vi "Transform.vi"(8 "error in (no error)":errorcluster, 9 "Offset":u64, 10 "Transformation Map":refnum<class "Range.lvclass">, 11 "Range in":refnum<class "Range.lvclass">) -> (0 "error out":errorcluster, 2 "Remainder":refnum<class "Range.lvclass">, 3 "Range out":refnum<class "Range.lvclass">)   [LabVIEW 2020, in "Range.lvclass"]
uses:
  Range.lvclass
  Range.lvclass/Range.ctl
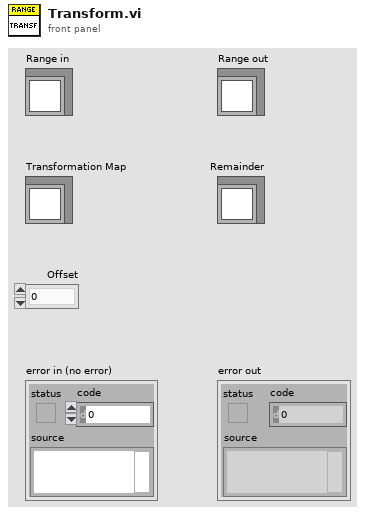
[diagram p1: front panel]
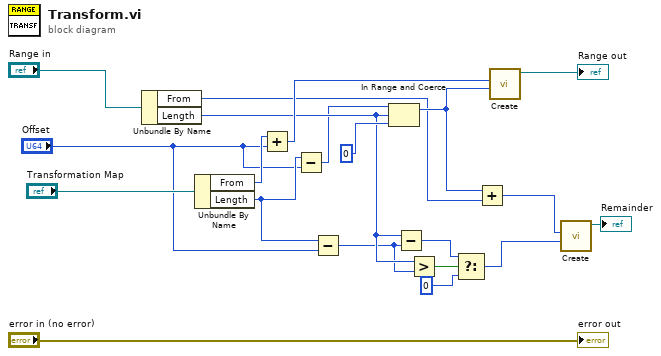
[diagram p0: block diagram]
diagram:
  n1 = Unbundle By Name("Range in") -> ("From"=w11:u64, "Length"=w8:u64)
  n2 = Unbundle By Name("Transformation Map") -> ("From"=w16:u64, "Length"=w13:u64)
  n3 = Add(x=w16, y="Offset") -> (x+y=w14:u64)
  n4 = Subtract(x=w13, y="Offset") -> (x-y=w2:u64)
  n5 = Subtract(x=w13, y="Offset") -> (x-y=w7:u64)
  n6 = In Range and Coerce(upper limit=w2, x=w8, lower limit=u64 0) -> (coerced(x)=w12:u64)  [unwired: 1 out]
  n7 = Subtract(x=w8, y=w7) -> (x-y=w5:u64)
  n8 = Greater?(x=w8, y=w7) -> (0:w6:bool)
  n9 = Select(t=w5, s=w6, f=u64 0) -> (s? t:f=w4:u64)
  n10 = Add(x=w12, y=w11) -> (x+y=w10:u64)
  n11 = call "Create.vi"("Length"=w12, "From"=w14) -> ("Range"=→"Range out":refnum<class "Range.lvclass">)  [unwired: 8 in, 1 out]
  n12 = call "Create.vi"("Length"=w4, "From"=w10) -> ("Range"=→"Remainder":refnum<class "Range.lvclass">)  [unwired: 8 in, 1 out]
  "error out" <- "error in (no error)"
